vi "daqhat_tcp_iepe.vi"(8 "error in (no error)":errorcluster, 9 "IEPE Power":bool, 10 "Channel":u8 max=1, 11 "TCP network connection in":refnum<k5>) -> (0 "error out":errorcluster, 3 "TCP Network Connection out":refnum<k5>)   [LabVIEW 2018]
doc: "Set MCC 172 IEPE power using a TCP server running on a Raspberry Pi. The TCP server program must be running on the Pi, and the TCP connection already opened to the correct IP address and port. Provide the frequency in Hz."
panel:
  out "String":string
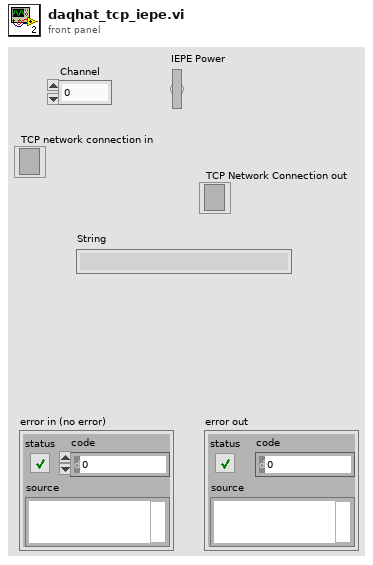
[diagram p1: front panel]
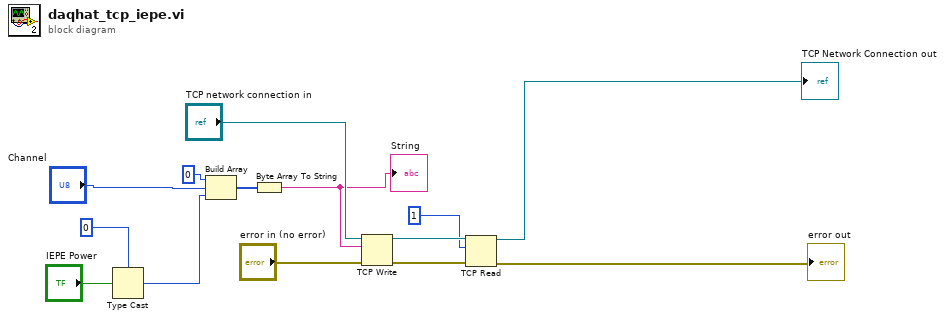
[diagram p0: block diagram]
diagram:
  n1 = Type Cast(type=u8 0, x="IEPE Power") -> (*(type *) &x=w6:u8)
  n2 = Build Array(u8 0, "Channel", w6) -> (w14:u8[])
  n3 = Byte Array To String(unsigned byte array=w14) -> (string=w10:string)
  "String" <- w10
  n4 = TCP Write(connection ID="TCP network connection in", data in=w10, error in (no error)="error in (no error)") -> (connection ID out=w5:refnum<k5>, error out=w4:errorcluster)  [unwired: 1 in, 1 out]
  n5 = TCP Read(connection ID=w5, bytes to read=1, error in (no error)=w4) -> (connection ID out=→"TCP Network Connection out":refnum<k5>, error out=→"error out":errorcluster)  [unwired: 2 in, 1 out]
